vi "SetTo0.vi"(10 "Longueur d'onde":dbl) -> (2 "Température 0":dbl)   [LabVIEW 2018]
uses:
  <vilib>/Analysis/NI_AALBase.lvlib
  <vilib>/Analysis/baseanly.llb/Mean (DBL).vi
  <vilib>/DAQmx/configure/timing.llb/DAQmx Timing (Sample Clock).vi
  <vilib>/DAQmx/create/channels.llb/DAQmx Create Channel (AI-Voltage-Basic).vi
  <vilib>/DAQmx/read.llb/DAQmx Read (Analog 1D Wfm NChan NSamp).vi
  <resource>/objmgr/daqmx.rc
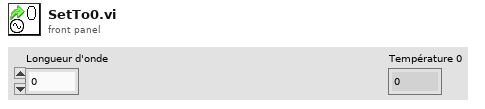
[diagram p1: front panel]
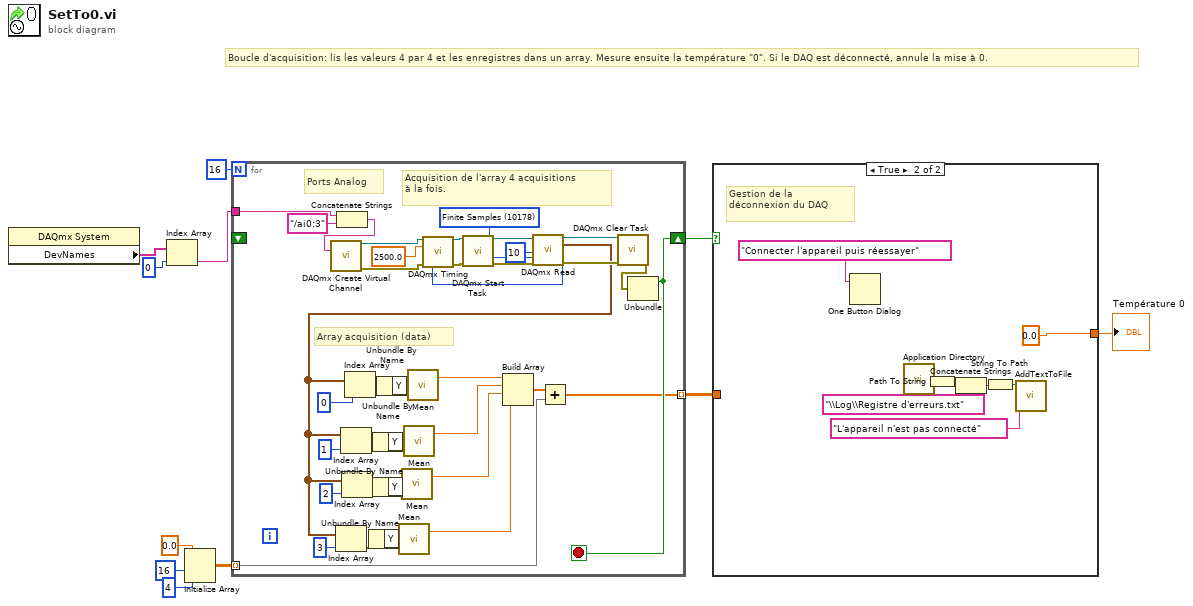
[diagram p0: block diagram]
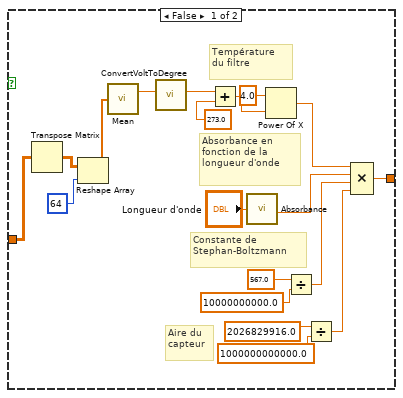
[diagram p2: hidden frame]
diagram:
  # "Boucle d'acquisition: lis les valeurs 4 par 4 et les enregistres dans un array. Mesure ensuite la température \"0\". Si le DAQ est déconnecté, annule la mise à 0."
  n1 = property class="DAQmx System"() -> ("DevNames"=w3:tag[])  [unwired: 2 in, 2 out]
  n2 = Index Array(array=w3, index=0) -> (element=w2:tag)
  n3 = Initialize Array(0.0 ("element"), 16 ("dimension size"), 4 ("dimension size")) -> (w6:dbl[][])
  n4 = for {
    N: 16 -> [_]
    shift-right: [w22] -> w10
    shift-left: _ -> [_]
    tunnel: w6 -> [w16] mode=indexing
    tunnel: [w15] -> w4 mode=indexing
    tunnel: w2 -> [w12]
    stop <- w22 stop-if-true
    w26 = 10178 items=["Finite Samples"=10178, "Continuous Samples"=10123, "Hardware Timed Single Point"=12522] ("sample mode")
    # "Ports Analog"
    # "Array acquisition (data)"
    # "Acquisition de l'array 4 acquisitions\nà la fois."
    n5 = Concatenate Strings(w12, "/ai0:3" ("string")) -> (w13:string)
    n6 = call-poly <vilib>:"DAQmx Create Virtual Channel.vi"("physical channels"=w13) -> ("task out"=w46:refnum<k21>, "error out"=w45:errorcluster)  [unwired: 13 in]
    n7 = call-poly <vilib>:"DAQmx Timing.vi"("task/channels in"=w46, "sample mode"=w26, "rate"=2500.0, "error in"=w45) -> ("task out"=w42:refnum<k21>, "error out"=w43:errorcluster)  [unwired: 10 in]
    n8 = call <vilib>:"DAQmx Start Task.vi"("task/channels in"=w42, "error in"=w43) -> ("task out"=w44:refnum<k21>, "error out"=w47:errorcluster)  [unwired: 12 in]
    n9 = call-poly <vilib>:"DAQmx Read.vi"("task/channels in"=w44, "number of samples per channel"=10, "error in"=w47) -> ("task out"=w32:refnum<k21>, "data"=w23:waveform(dbl)[], "error out"=w31:errorcluster)  [unwired: 10 in]
    n10 = Index Array(array=w23, index=3) -> (element=w37:waveform(dbl))
    n11 = Index Array(array=w23, index=1) -> (element=w39:waveform(dbl))
    n12 = Index Array(array=w23, index=2) -> (element=w38:waveform(dbl))
    n13 = Index Array(array=w23, index=0) -> (element=w40:waveform(dbl))
    n14 = Unbundle By Name(w37) -> ("Y"=w33:dbl[])
    n15 = Unbundle By Name(w39) -> ("Y"=w35:dbl[])
    n16 = Unbundle By Name(w38) -> ("Y"=w34:dbl[])
    n17 = Unbundle By Name(w40) -> ("Y"=w36:dbl[])
    n18 = call-poly <vilib>:"Mean.vi"("X"=w33) -> ("mean"=w18:dbl)  [unwired: 1 out]
    n19 = call-poly <vilib>:"Mean.vi"("X"=w34) -> ("mean"=w19:dbl)  [unwired: 1 out]
    n20 = call-poly <vilib>:"Mean.vi"("X"=w35) -> ("mean"=w20:dbl)  [unwired: 1 out]
    n21 = call-poly <vilib>:"Mean.vi"("X"=w36) -> ("mean"=w21:dbl)  [unwired: 1 out]
    n22 = Build Array(w21, w20, w19, w18) -> (w17:dbl[])
    n23 = Add(x=w17, y=w16) -> (x+y=w15:dbl[])
    n24 = call <vilib>:"DAQmx Clear Task.vi"("task in"=w32, "error in"=w31) -> ("error out"=w41:errorcluster)  [unwired: 13 in]
    n25 = Unbundle(w41) -> ("status"=w22:bool)  [unwired: 2 out]
  }
  n26 = case shown="True" w10 {
    tunnel: w4 -> [w52 _]
    tunnel: [w48 0.0] -> w5
    frame False {
      # "Constante de \nStephan-Boltzmann"
      # "Absorbance en\nfonction de la \nlongueur d'onde"
      # "Température \ndu filtre"
      # "Aire du\ncapteur"
      n27 = Transpose Matrix(1:w52) -> (0:w53:dbl[][])
      n28 = Reshape Array(w53, 64 ("dimension size")) -> (w50:dbl[])
      n29 = call-poly <vilib>:"Mean.vi"("X"=w50) -> ("mean"=w49:dbl)  [unwired: 1 out]
      n30 = call "ConvertVoltToDegree.vi"("Tension"=w49) -> ("Température"=w58:dbl)  [unwired: 10 in]
      n31 = Add(x=w58, y=273.0) -> (x+y=w65:dbl)
      n32 = call "Absorbance.vi"("Longueur d'onde"="Longueur d'onde") -> ("absorbance"=w55:dbl)  [unwired: 10 in]
      n33 = Power Of X(1:w65, 2:4.0 ("y")) -> (0:w54:dbl)
      n34 = Divide(x=567.0, y=10000000000.0) -> (x/y=w56:dbl)
      n35 = Divide(x=2026829916.0, y=1000000000000.0) -> (x/y=w57:dbl)
      n36 = Compound Arithmetic op=MULTIPLY(w54, w55, w56, w57) -> (w48:dbl)
    }
    frame True {
      # "Gestion de la \ndéconnexion du DAQ"
      n37 = One Button Dialog(message="Connecter l'appareil puis réessayer") -> ()  [unwired: 1 in, 1 out]
      n38 = call <vilib>:"Application Directory.vi"() -> ("Application Directory"=w70:path)
      n39 = Path To String(path=w70) -> (string=w71:string)
      n40 = Concatenate Strings(w71, "\\Log\\Registre d'erreurs.txt") -> (w72:string)
      n41 = String To Path(string=w72) -> (path=w68:path)
      n42 = call "AddTextToFile.vi"("Ajouter du texte"="L'appareil n'est pas connecté", "Fichier"=w68) -> ()  [unwired: 10 in]
    }
  }
  "Température 0" <- w5
